vi "TXSIG_Generate(SubVi).vi"(5 "Chip_rate_Threshold":dbl=5.0 format="%#_13g", 7 "ThresHold":dbl=5.0 format="%#_13g", 8 "Version 스위치":bool, 9 "Rc":dbl=5500.0 format="%#_13g", 10 "길이":i32=256, 11 "이름 또는 상대 경로":string) -> (1 "TXN":dbl[](array[numeric]), 2 "TXP":dbl[](array[numeric]), 4 "TXSIG":waveform(dbl)[](graph))   [LabVIEW 2017]
uses:
  <vilib>/Analysis/NI_AALBase.lvlib
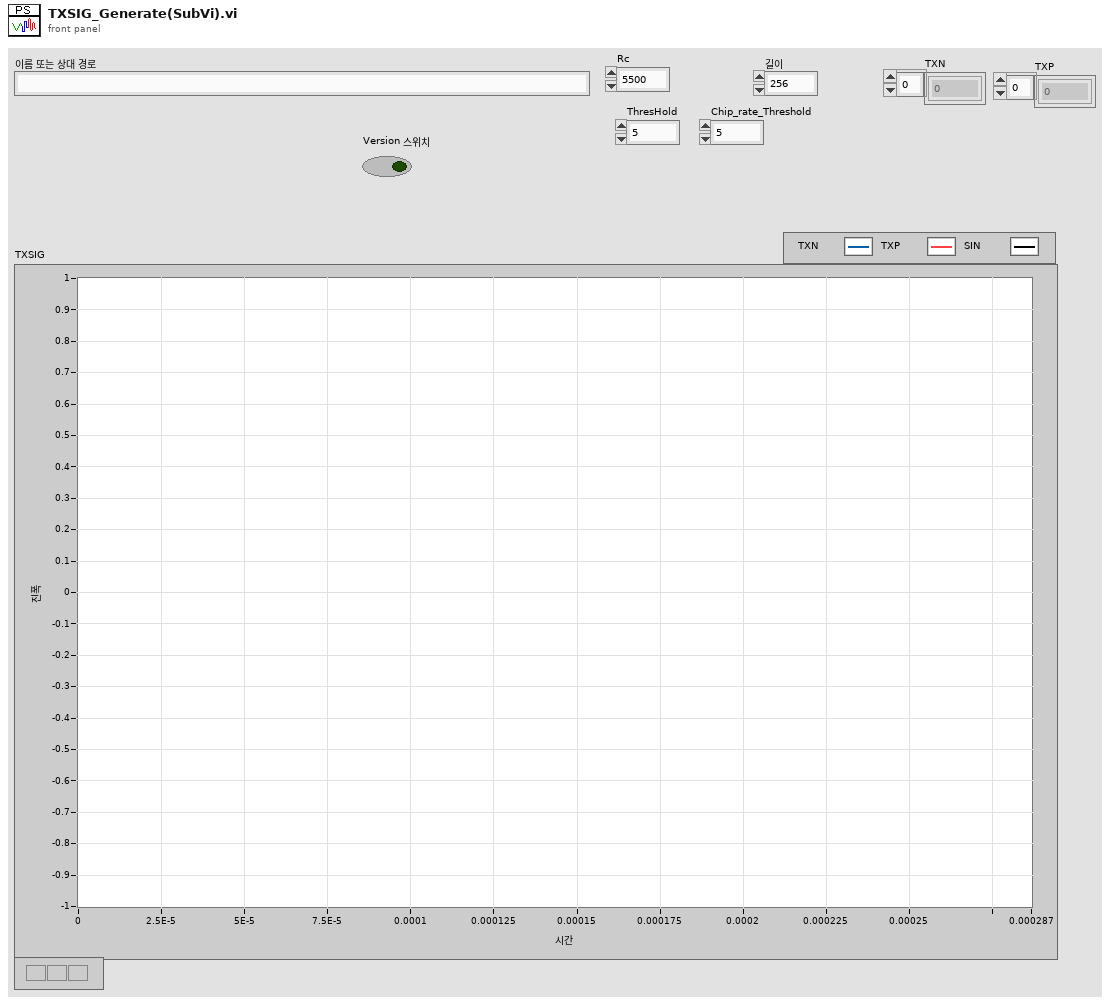
[diagram p1: front panel]
types:
  T1 = enum16{"open", "open or create", "create or replace", "create", "open (read-only)"}
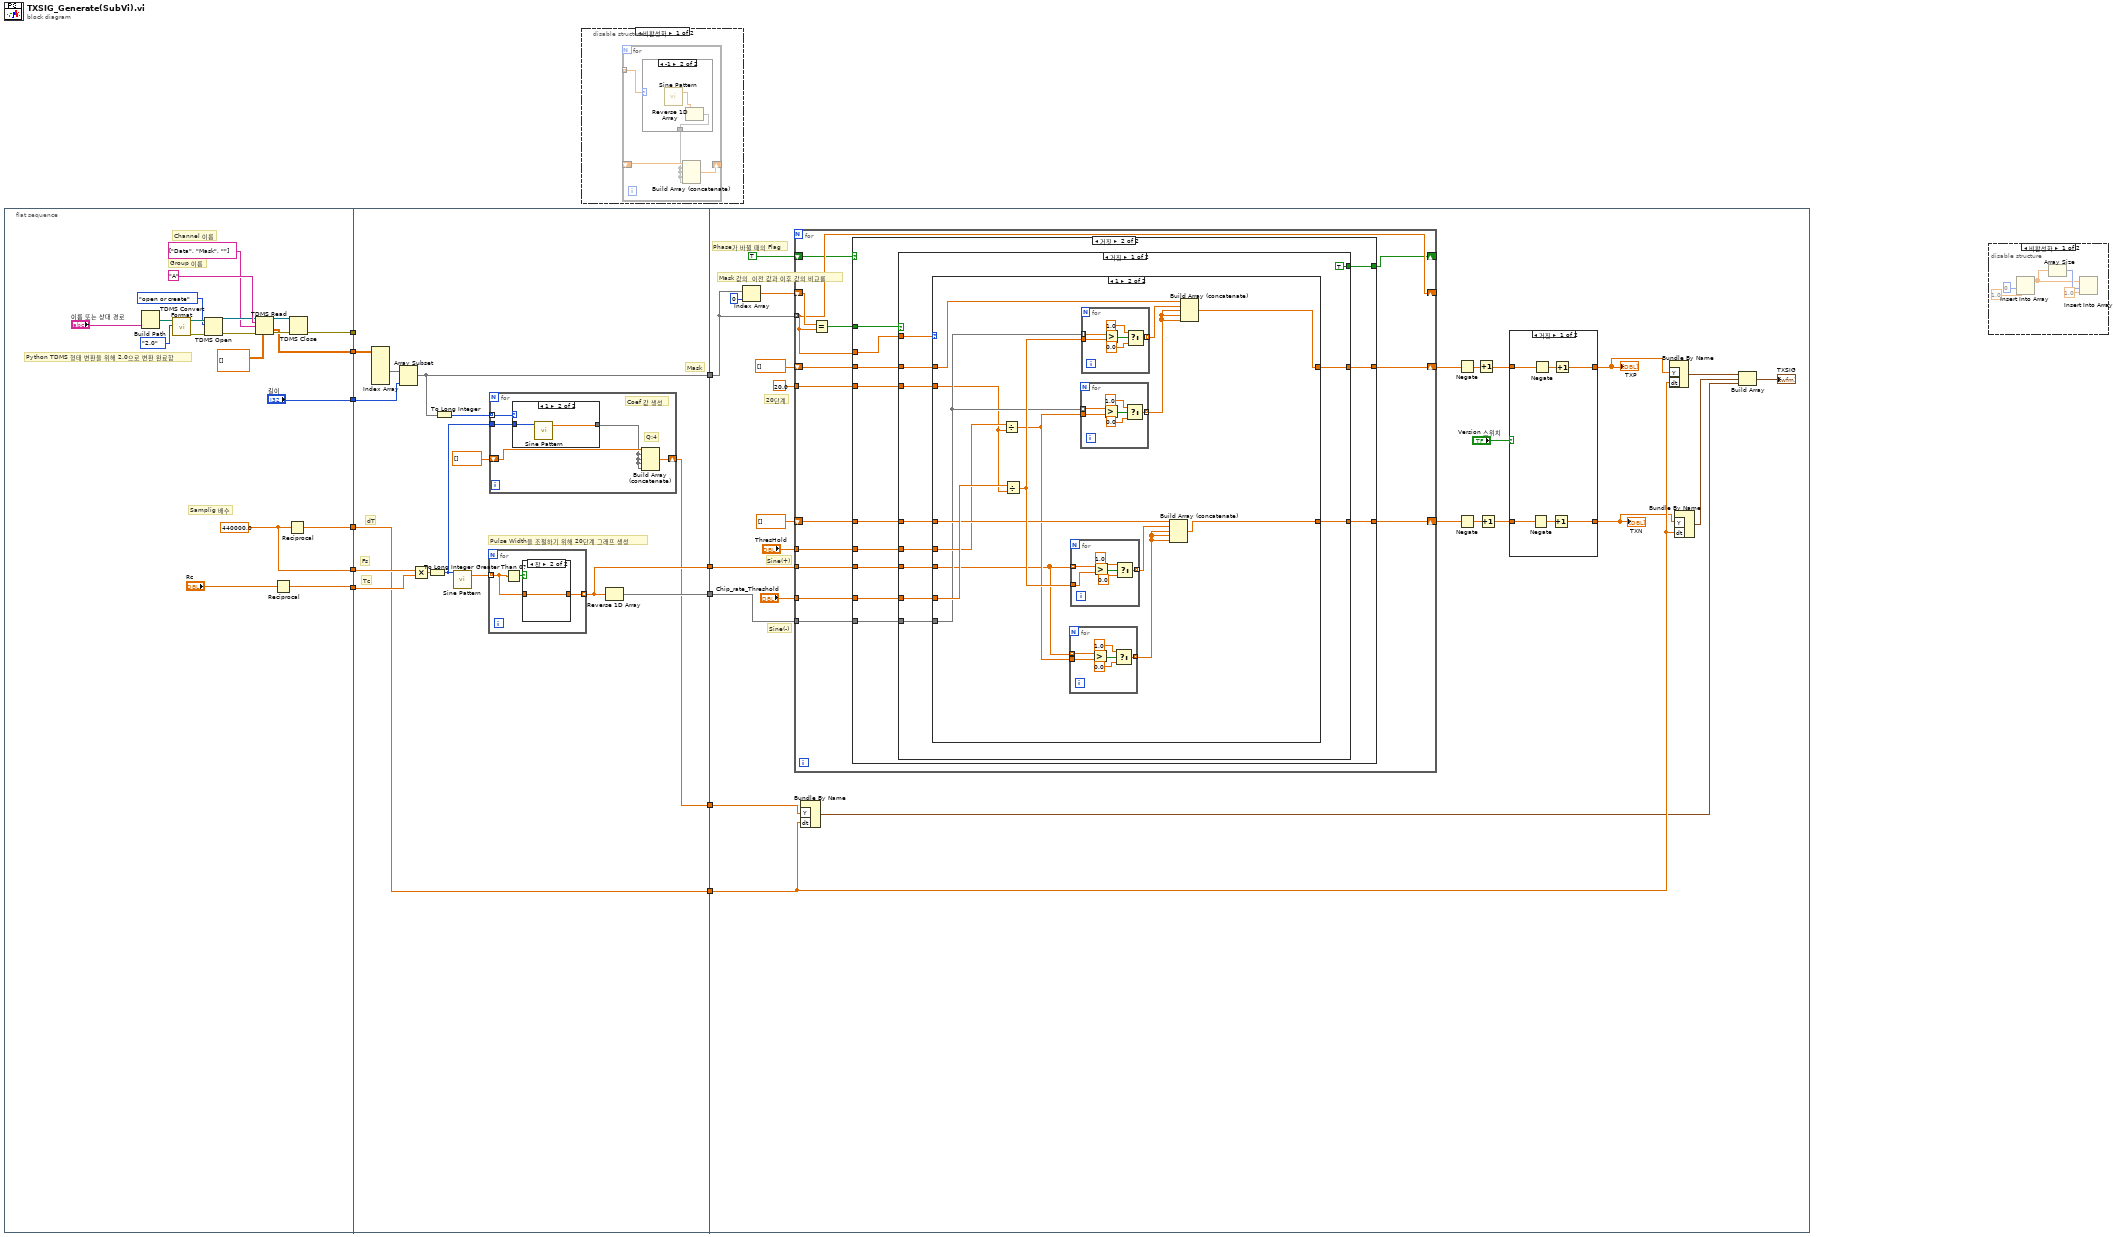
[diagram p0: block diagram]
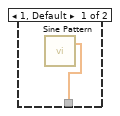
[diagram p2: hidden frame]
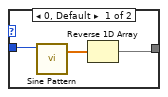
[diagram p5: hidden frame]
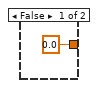
[diagram p6: hidden frame]
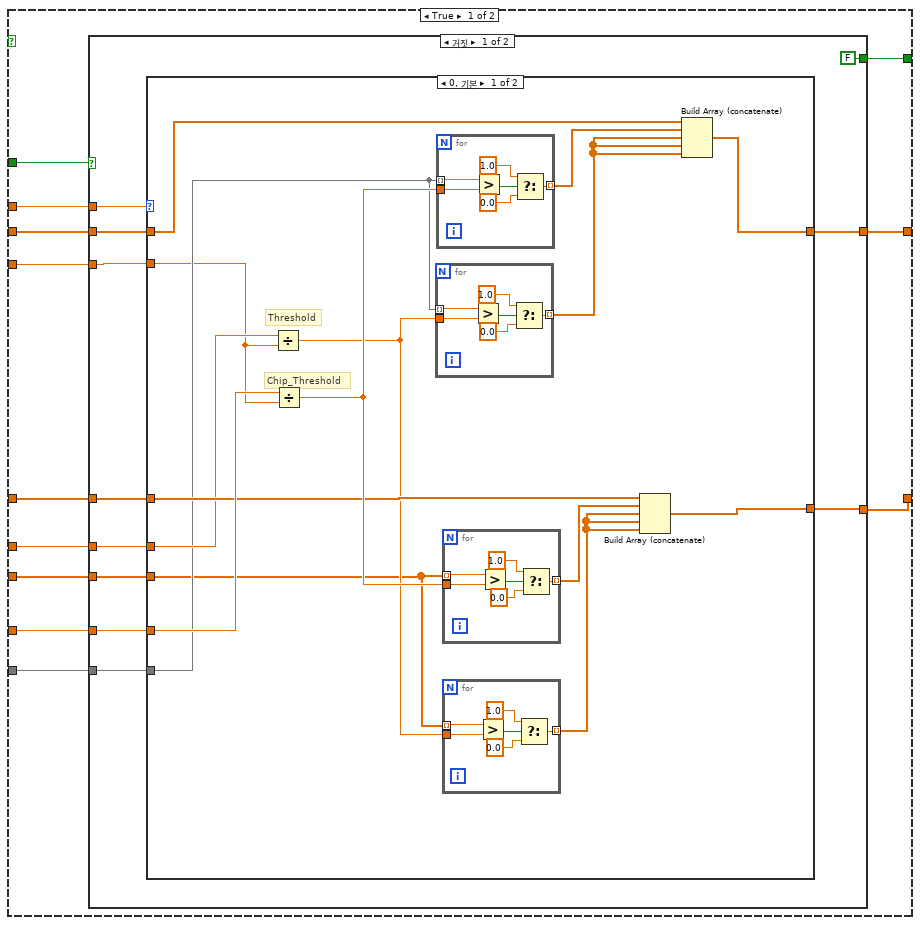
[diagram p8: hidden frame]
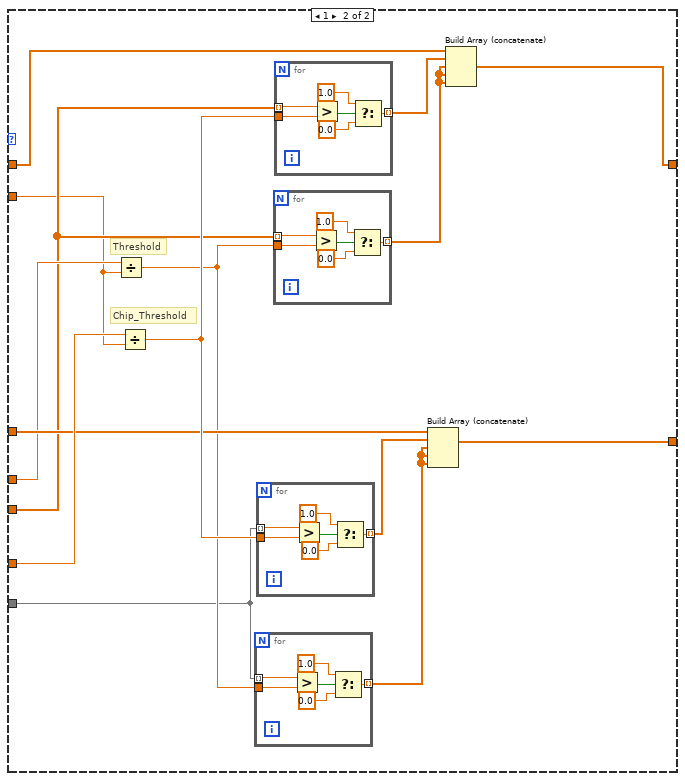
[diagram p9: hidden frame]
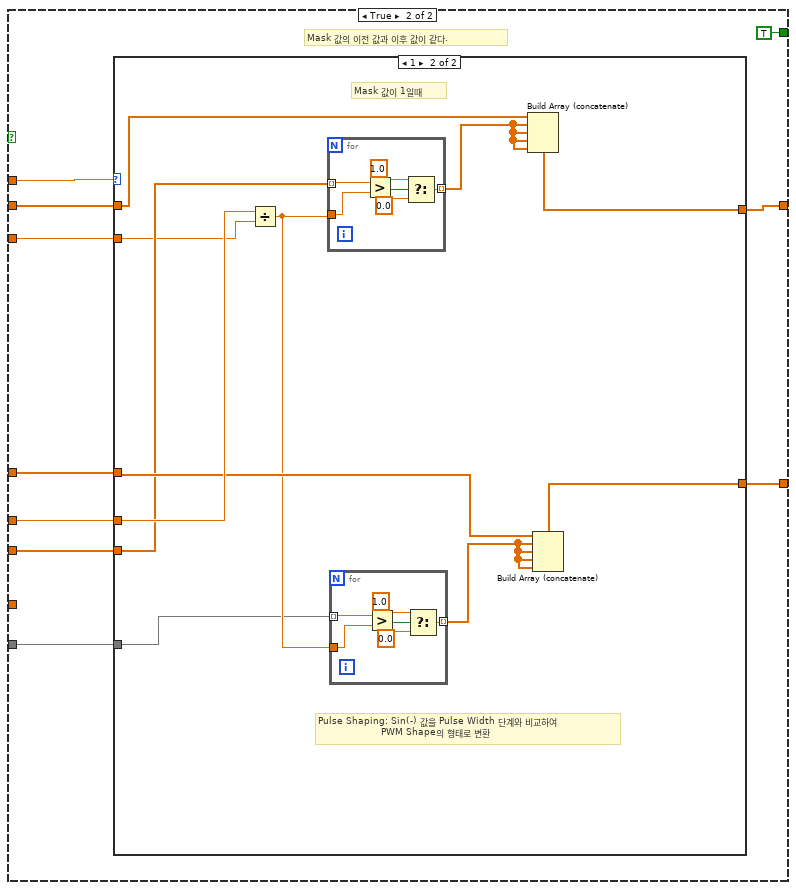
[diagram p10: hidden frame]
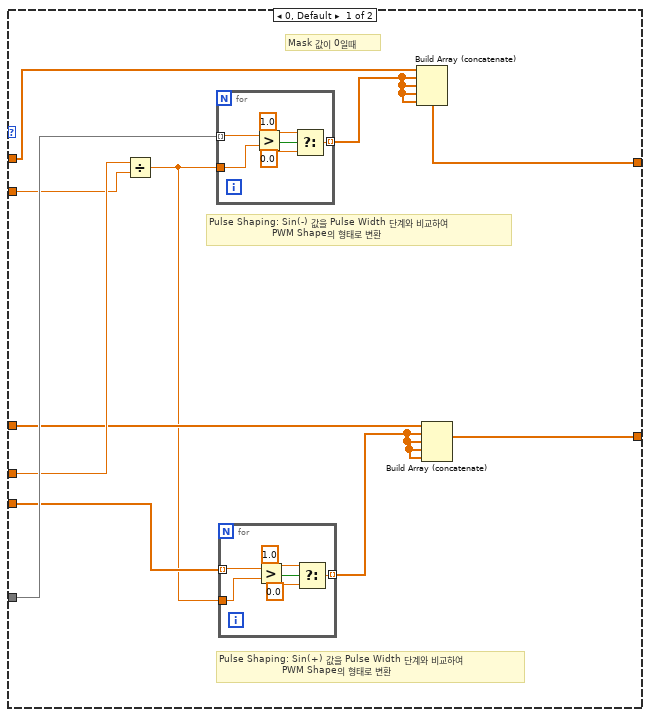
[diagram p11: hidden frame]
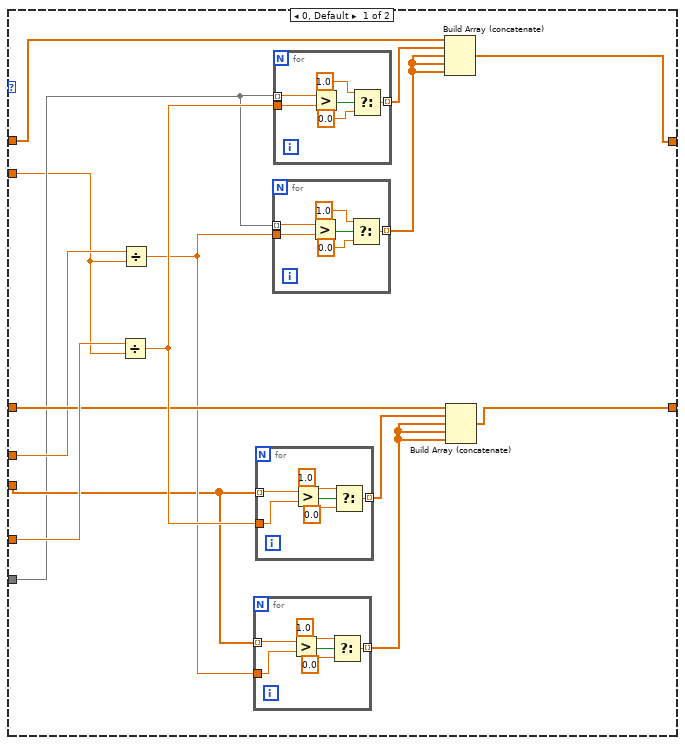
[diagram p12: hidden frame]
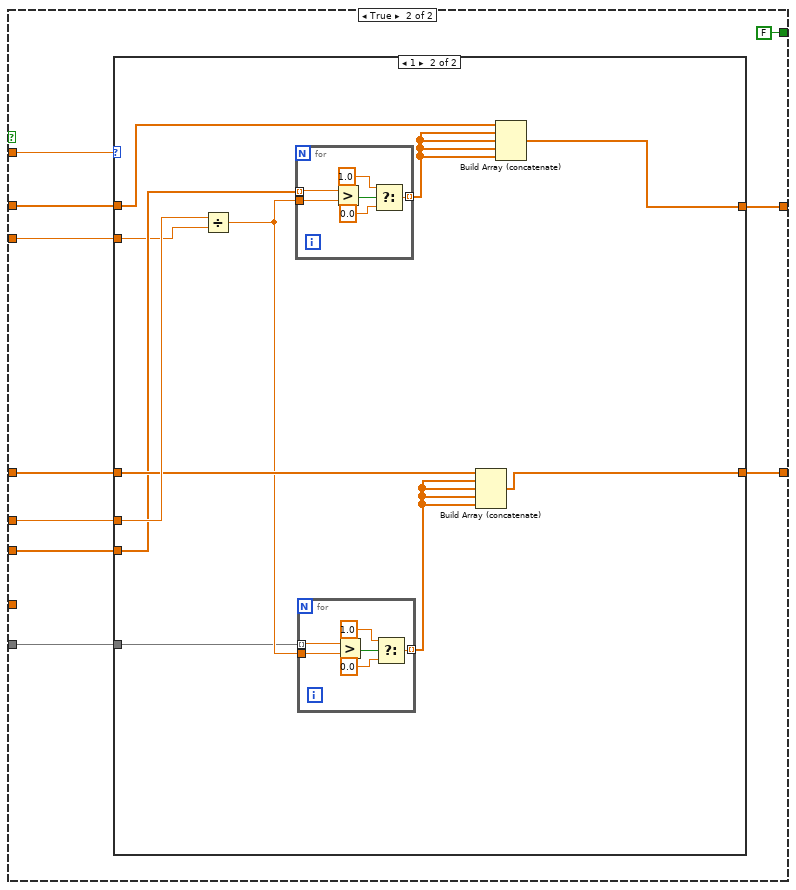
[diagram p13: hidden frame]
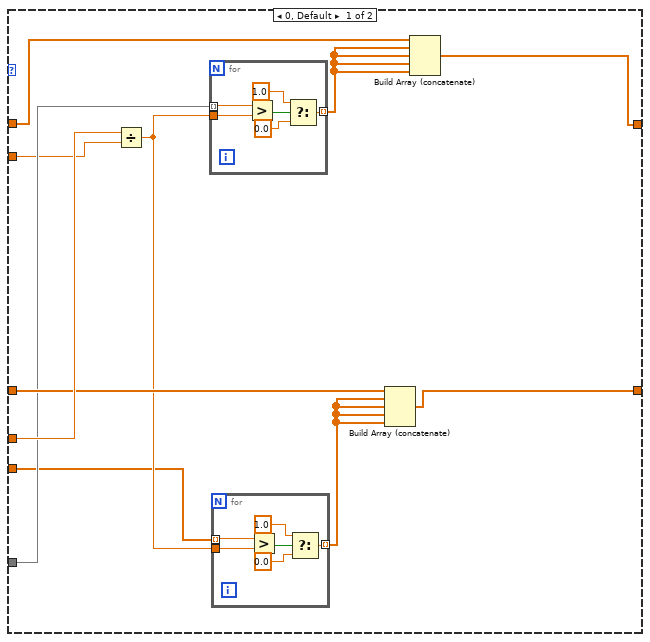
[diagram p14: hidden frame]
diagram:
  n1 = flat-sequence {
    tunnel: [w20] -> w11
    tunnel: [w19] -> w10
    tunnel: ["길이"] -> w6
    tunnel: [w13] -> w5
    tunnel: [w12] -> w4
    tunnel: [w15] -> w3
    tunnel: w10 -> [_]
    tunnel: w11 -> [w43]
    tunnel: [w38] -> w9
    tunnel: [w35] -> w8
    tunnel: [w45] -> w7
    tunnel: w6 -> [w42]
    tunnel: w5 -> [w40]
    tunnel: w4 -> [w39]
    tunnel: w3 -> [w32]
    tunnel: [w34] -> w2
    tunnel: [w32] -> w1
    tunnel: w9 -> [w86]
    tunnel: w8 -> [w83]
    tunnel: w7 -> [w80]
    tunnel: w2 -> [w67]
    tunnel: w1 -> [w72]
    frame #0 {
      w12 = 440000.0
      # "Samplig 배수"
      # "Python TDMS 형태 변환을 위해 2.0으로 변환 완료함"
      # "Group 이름"
      # "Channel 이름"
      n2 = Build Path(name or relative path="이름 또는 상대 경로") -> (appended path=w30:path)  [unwired: 1 in]
      n3 = call <vilib>:"TDMS Convert Format.vi"("target version"=enum16{"1.0", "2.0"}."2.0", "file path"=w30) -> ("error out"=w25:errorcluster, "file path out"=w24:path)  [unwired: 4 in]
      n4 = TDMS Open(8:w25, 10:T1."open or create" ("operation (0:open)"), 11:w24) -> (0:w21:errorcluster, 3:w22:refnum<k34>)  [unwired: 4 in]
      n5 = TDMS Read(0:w22, 5:"A" ("그룹 이름 입력"), 7:string[] ["Data", "Mask", ""] ("채널 이름 입력"), 11:w21, 12:dbl[][] []) -> (4:w27:refnum<k34>, 10:w20:dbl[][], 15:w26:errorcluster)  [unwired: 3 in, 3 out]
      n6 = Reciprocal(x="Rc") -> (1/x=w13:dbl)
      n7 = Reciprocal(x=w12) -> (1/x=w15:dbl)
      n8 = TDMS Close(8:w26, 11:w27) -> (0:w19:errorcluster)  [unwired: 1 out]
    }
    frame #1 {
      # "dT"
      # "Mask"
      # "Pulse Width을 조절하기 위해 20단계 그래프 생성"
      # "Tc"
      # "Fs"
      n9 = Index Array(array=w43) -> (element #2=w44:dbl[])  [unwired: 6 in, 2 out]
      n10 = Array Subset(array=w44, length=w42) -> (w38:dbl[])  [unwired: 1 in]
      n11 = Multiply(x=w39, y=w40) -> (x*y=w41:dbl)
      n12 = To Long Integer(number=w41) -> (32bit integer=w33:i32)
      n13 = To Long Integer(number=w38) -> (32bit integer=w37:i32[])
      n14 = call <vilib>:"Sine Pattern.vi"("samples"=w33) -> ("Sinusoidal Pattern"=w46:dbl[])  [unwired: 3 in, 1 out]
      n15 = for {
        tunnel: w46 -> [w58] mode=indexing
        tunnel: [w57] -> w35 mode=indexing
        n16 = Greater Than 0?(x=w58) -> (x > 0?=w59:bool)
        n17 = case shown="참" w59 {
          tunnel: w58 -> [_ w61]
          tunnel: [0.0 w61] -> w57
          frame False {
          }
          frame True {
          }
        }
      }
      n18 = for {
        tunnel: w33 -> [w51]
        tunnel: w37 -> [w50] mode=indexing
        shift-right: [w47] -> w34
        shift-left: dbl[] [] -> [w49]
        # "Coef 값 생성"
        # "Q:4"
        n19 = case shown="1" w50 {
          tunnel: [w52 w55] -> w48
          tunnel: w51 -> [w54 w56]
          frame 0, Default {
            n20 = call <vilib>:"Sine Pattern.vi"("samples"=w54) -> ("Sinusoidal Pattern"=w53:dbl[])  [unwired: 3 in, 1 out]
            n21 = Reverse 1D Array(array=w53) -> (reversed array=w52:dbl[])
          }
          frame 1 {
            n22 = call <vilib>:"Sine Pattern.vi"("samples"=w56) -> ("Sinusoidal Pattern"=w55:dbl[])  [unwired: 3 in, 1 out]
          }
        }
        n23 = Build Array (concatenate)(w49, w48, w48, w48, w48) -> (w47:dbl[])
      }
      n24 = Reverse 1D Array(array=w35) -> (reversed array=w45:dbl[])
    }
    frame #2 {
      # "20단계"
      # "Mask 값의  이전 값과 이후 값의 비교를"
      # "Phase가 바뀔 때의 Flag"
      # "Sine(-)"
      # "Sine(+)"
      n25 = Index Array(array=w86, index=0 ("인덱스")) -> (element=w84:dbl)
      n26 = for {
        shift-right: [w97] -> _
        shift-left: TRUE -> [w98]
        tunnel: w86 -> [w107] mode=indexing
        shift-right: [w107] -> _
        shift-left: w84 -> [w109]
        tunnel: w83 -> [w106]
        shift-right: [w102] -> w77
        shift-left: dbl[] [] -> [w104]
        shift-right: [w101] -> w76
        shift-left: dbl[] [] -> [w105]
        tunnel: w80 -> [w103]
        tunnel: "ThresHold" -> [w100]
        tunnel: "Chip_rate_Threshold" -> [w99]
        tunnel: 20.0 ("y") -> [w96]
        n27 = Equal?(x=w109, y=w107) -> (x = y?=w108:bool)
        n28 = case shown="거짓" w98 {
          tunnel: w108 -> [w121 w278]
          tunnel: w107 -> [w120 w277]
          tunnel: w106 -> [w119 w276]
          tunnel: w105 -> [w118 w275]
          tunnel: w104 -> [w117 w274]
          tunnel: w103 -> [w116 w273]
          tunnel: [w115 w272] -> w102
          tunnel: [w114 w271] -> w101
          tunnel: w100 -> [w113 w270]
          tunnel: w99 -> [w112 w269]
          tunnel: [w111 w268] -> w97
          tunnel: w96 -> [w110 w267]
          frame True {
            n29 = case shown="거짓" w121 {
              tunnel: w120 -> [w132 w220]
              tunnel: w119 -> [w128 w216]
              tunnel: w118 -> [w130 w219]
              tunnel: w117 -> [w131 w218]
              tunnel: w116 -> [w127 w217]
              tunnel: [w125 w215] -> w115
              tunnel: [w124 w214] -> w114
              tunnel: w113 -> [w129 w213]
              tunnel: w112 -> [w126 _]
              tunnel: [FALSE TRUE] -> w111
              tunnel: w110 -> [w122 w211]
              frame False {
                n30 = case shown="0, 기본" w132 {
                  tunnel: w131 -> [w147 w186]
                  tunnel: w130 -> [w143 w182]
                  tunnel: w129 -> [w139 w178]
                  tunnel: w128 -> [w135 w174]
                  tunnel: w127 -> [w138 w173]
                  tunnel: w126 -> [w146 w185]
                  tunnel: [w145 w184] -> w125
                  tunnel: [w142 w181] -> w124
                  tunnel: w122 -> [w133 w172]
                  frame 0, Default {
                    # "Threshold"
                    # "Chip_Threshold"
                    n31 = Divide(x=w139, y=w133) -> (x/y=w136:dbl)
                    n32 = Divide(x=w146, y=w133) -> (x/y=w144:dbl)
                    n33 = for {
                      tunnel: w138 -> [w159] mode=indexing
                      tunnel: w136 -> [w158]
                      tunnel: [w154] -> w137 mode=indexing
                      n34 = Greater?(x=w159, y=w158) -> (0:w157:bool)
                      n35 = Select(t=1.0, s=w157, f=0.0) -> (s? t:f=w154:dbl)
                    }
                    n36 = for {
                      tunnel: w138 -> [w171] mode=indexing
                      tunnel: w144 -> [w170]
                      tunnel: [w166] -> w141 mode=indexing
                      n37 = Greater?(x=w171, y=w170) -> (0:w169:bool)
                      n38 = Select(t=1.0, s=w169, f=0.0) -> (s? t:f=w166:dbl)
                    }
                    n39 = for {
                      tunnel: w135 -> [w165] mode=indexing
                      tunnel: w144 -> [w164]
                      tunnel: [w160] -> w140 mode=indexing
                      n40 = Greater?(x=w165, y=w164) -> (0:w163:bool)
                      n41 = Select(t=1.0, s=w163, f=0.0) -> (s? t:f=w160:dbl)
                    }
                    n42 = for {
                      tunnel: w135 -> [w153] mode=indexing
                      tunnel: w136 -> [w152]
                      tunnel: [w148] -> w134 mode=indexing
                      n43 = Greater?(x=w153, y=w152) -> (0:w151:bool)
                      n44 = Select(t=1.0, s=w151, f=0.0) -> (s? t:f=w148:dbl)
                    }
                    n45 = Build Array (concatenate)(w143, w140, w134, w134, w134) -> (w142:dbl[])
                    n46 = Build Array (concatenate)(w147, w141, w137, w137, w137) -> (w145:dbl[])
                  }
                  frame 1 {
                    # "Chip_Threshold"
                    # "Threshold"
                    n47 = Divide(x=w178, y=w172) -> (x/y=w176:dbl)
                    n48 = Divide(x=w185, y=w172) -> (x/y=w183:dbl)
                    n49 = for {
                      tunnel: w173 -> [w192] mode=indexing
                      tunnel: w176 -> [w191]
                      tunnel: [w187] -> w175 mode=indexing
                      n50 = Greater?(x=w192, y=w191) -> (0:w190:bool)
                      n51 = Select(t=1.0, s=w190, f=0.0) -> (s? t:f=w187:dbl)
                    }
                    n52 = for {
                      tunnel: w173 -> [w204] mode=indexing
                      tunnel: w183 -> [w203]
                      tunnel: [w199] -> w179 mode=indexing
                      n53 = Greater?(x=w204, y=w203) -> (0:w202:bool)
                      n54 = Select(t=1.0, s=w202, f=0.0) -> (s? t:f=w199:dbl)
                    }
                    n55 = for {
                      tunnel: w174 -> [w198] mode=indexing
                      tunnel: w176 -> [w197]
                      tunnel: [w193] -> w177 mode=indexing
                      n56 = Greater?(x=w198, y=w197) -> (0:w196:bool)
                      n57 = Select(t=1.0, s=w196, f=0.0) -> (s? t:f=w193:dbl)
                    }
                    n58 = for {
                      tunnel: w174 -> [w210] mode=indexing
                      tunnel: w183 -> [w209]
                      tunnel: [w205] -> w180 mode=indexing
                      n59 = Greater?(x=w210, y=w209) -> (0:w208:bool)
                      n60 = Select(t=1.0, s=w208, f=0.0) -> (s? t:f=w205:dbl)
                    }
                    n61 = Build Array (concatenate)(w182, w179, w175, w175, w175) -> (w181:dbl[])
                    n62 = Build Array (concatenate)(w186, w180, w177, w177, w177) -> (w184:dbl[])
                  }
                }
              }
              frame True {
                # "Mask 값의 이전 값과 이후 값이 같다."
                n63 = case shown="1" w220 {
                  tunnel: w219 -> [w227 w251]
                  tunnel: w218 -> [w231 w254]
                  tunnel: w217 -> [w229 w246]
                  tunnel: w216 -> [w226 w245]
                  tunnel: [w230 w253] -> w215
                  tunnel: [w224 w249] -> w214
                  tunnel: w213 -> [w228 w252]
                  tunnel: w211 -> [w221 w244]
                  frame 0, Default {
                    # "Pulse Shaping: Sin(+) 값을 Pulse Width 단계와 비교하여\n                     PWM Shape의 형태로 변환"
                    # "Pulse Shaping: Sin(-) 값을 Pulse Width 단계와 비교하여\n                     PWM Shape의 형태로 변환"
                    # "Mask 값이 0일때"
                    n64 = Divide(x=w228, y=w221) -> (x/y=w225:dbl)
                    n65 = for {
                      tunnel: w229 -> [w243] mode=indexing
                      tunnel: w225 -> [w242]
                      tunnel: [w238] -> w223 mode=indexing
                      n66 = Greater?(x=w243, y=w242) -> (0:w241:bool)
                      n67 = Select(t=1.0, s=w241, f=0.0) -> (s? t:f=w238:dbl)
                    }
                    n68 = for {
                      tunnel: w226 -> [w237] mode=indexing
                      tunnel: w225 -> [w236]
                      tunnel: [w232] -> w222 mode=indexing
                      n69 = Greater?(x=w237, y=w236) -> (0:w235:bool)
                      n70 = Select(t=1.0, s=w235, f=0.0) -> (s? t:f=w232:dbl)
                    }
                    n71 = Build Array (concatenate)(w231, w223, w223, w223, w223) -> (w230:dbl[])
                    n72 = Build Array (concatenate)(w227, w222, w222, w222, w222) -> (w224:dbl[])
                  }
                  frame 1 {
                    # "Pulse Shaping: Sin(-) 값을 Pulse Width 단계와 비교하여\n                     PWM Shape의 형태로 변환"
                    # "Mask 값이 1일때"
                    n73 = Divide(x=w252, y=w244) -> (x/y=w250:dbl)
                    n74 = for {
                      tunnel: w245 -> [w266] mode=indexing
                      tunnel: w250 -> [w265]
                      tunnel: [w261] -> w248 mode=indexing
                      n75 = Greater?(x=w266, y=w265) -> (0:w264:bool)
                      n76 = Select(t=1.0, s=w264, f=0.0) -> (s? t:f=w261:dbl)
                    }
                    n77 = for {
                      tunnel: w246 -> [w260] mode=indexing
                      tunnel: w250 -> [w259]
                      tunnel: [w255] -> w247 mode=indexing
                      n78 = Greater?(x=w260, y=w259) -> (0:w258:bool)
                      n79 = Select(t=1.0, s=w258, f=0.0) -> (s? t:f=w255:dbl)
                    }
                    n80 = Build Array (concatenate)(w254, w248, w248, w248, w248) -> (w253:dbl[])
                    n81 = Build Array (concatenate)(w251, w247, w247, w247, w247) -> (w249:dbl[])
                  }
                }
              }
            }
          }
          frame False {
            n82 = case shown="거짓" w278 {
              tunnel: w277 -> [w289 w377]
              tunnel: w276 -> [w285 w373]
              tunnel: w275 -> [w287 w376]
              tunnel: w274 -> [w288 w375]
              tunnel: w273 -> [w284 w374]
              tunnel: [w282 w372] -> w272
              tunnel: [w281 w371] -> w271
              tunnel: w270 -> [w286 w370]
              tunnel: w269 -> [w283 _]
              tunnel: [TRUE FALSE] -> w268
              tunnel: w267 -> [w279 w368]
              frame False {
                n83 = case shown="1" w289 {
                  tunnel: w288 -> [w304 w343]
                  tunnel: w287 -> [w300 w339]
                  tunnel: w286 -> [w296 w335]
                  tunnel: w285 -> [w293 w330]
                  tunnel: w284 -> [w292 w331]
                  tunnel: w283 -> [w303 w342]
                  tunnel: [w302 w341] -> w282
                  tunnel: [w299 w338] -> w281
                  tunnel: w279 -> [w291 w329]
                  frame 0, Default {
                    n84 = Divide(x=w303, y=w291) -> (x/y=w301:dbl)
                    n85 = Divide(x=w296, y=w291) -> (x/y=w294:dbl)
                    n86 = for {
                      tunnel: w293 -> [w310] mode=indexing
                      tunnel: w294 -> [w309]
                      tunnel: [w305] -> w290 mode=indexing
                      n87 = Greater?(x=w310, y=w309) -> (0:w308:bool)
                      n88 = Select(t=1.0, s=w308, f=0.0) -> (s? t:f=w305:dbl)
                    }
                    n89 = for {
                      tunnel: w293 -> [w322] mode=indexing
                      tunnel: w301 -> [w321]
                      tunnel: [w317] -> w297 mode=indexing
                      n90 = Greater?(x=w322, y=w321) -> (0:w320:bool)
                      n91 = Select(t=1.0, s=w320, f=0.0) -> (s? t:f=w317:dbl)
                    }
                    n92 = for {
                      tunnel: w292 -> [w316] mode=indexing
                      tunnel: w294 -> [w315]
                      tunnel: [w311] -> w295 mode=indexing
                      n93 = Greater?(x=w316, y=w315) -> (0:w314:bool)
                      n94 = Select(t=1.0, s=w314, f=0.0) -> (s? t:f=w311:dbl)
                    }
                    n95 = for {
                      tunnel: w292 -> [w328] mode=indexing
                      tunnel: w301 -> [w327]
                      tunnel: [w323] -> w298 mode=indexing
                      n96 = Greater?(x=w328, y=w327) -> (0:w326:bool)
                      n97 = Select(t=1.0, s=w326, f=0.0) -> (s? t:f=w323:dbl)
                    }
                    n98 = Build Array (concatenate)(w304, w298, w295, w295, w295) -> (w302:dbl[])
                    n99 = Build Array (concatenate)(w300, w297, w290, w290, w290) -> (w299:dbl[])
                  }
                  frame 1 {
                    n100 = Divide(x=w335, y=w329) -> (x/y=w333:dbl)
                    n101 = Divide(x=w342, y=w329) -> (x/y=w340:dbl)
                    n102 = for {
                      tunnel: w330 -> [w349] mode=indexing
                      tunnel: w333 -> [w348]
                      tunnel: [w344] -> w332 mode=indexing
                      n103 = Greater?(x=w349, y=w348) -> (0:w347:bool)
                      n104 = Select(t=1.0, s=w347, f=0.0) -> (s? t:f=w344:dbl)
                    }
                    n105 = for {
                      tunnel: w330 -> [w361] mode=indexing
                      tunnel: w340 -> [w360]
                      tunnel: [w356] -> w336 mode=indexing
                      n106 = Greater?(x=w361, y=w360) -> (0:w359:bool)
                      n107 = Select(t=1.0, s=w359, f=0.0) -> (s? t:f=w356:dbl)
                    }
                    n108 = for {
                      tunnel: w331 -> [w355] mode=indexing
                      tunnel: w333 -> [w354]
                      tunnel: [w350] -> w334 mode=indexing
                      n109 = Greater?(x=w355, y=w354) -> (0:w353:bool)
                      n110 = Select(t=1.0, s=w353, f=0.0) -> (s? t:f=w350:dbl)
                    }
                    n111 = for {
                      tunnel: w331 -> [w367] mode=indexing
                      tunnel: w340 -> [w366]
                      tunnel: [w362] -> w337 mode=indexing
                      n112 = Greater?(x=w367, y=w366) -> (0:w365:bool)
                      n113 = Select(t=1.0, s=w365, f=0.0) -> (s? t:f=w362:dbl)
                    }
                    n114 = Build Array (concatenate)(w339, w336, w332, w332, w332) -> (w338:dbl[])
                    n115 = Build Array (concatenate)(w343, w337, w334, w334, w334) -> (w341:dbl[])
                  }
                }
              }
              frame True {
                n116 = case shown="1" w377 {
                  tunnel: w376 -> [w385 w408]
                  tunnel: w375 -> [w388 w411]
                  tunnel: w374 -> [w380 w403]
                  tunnel: w373 -> [w379 w402]
                  tunnel: [w387 w410] -> w372
                  tunnel: [w383 w406] -> w371
                  tunnel: w370 -> [w386 w409]
                  tunnel: w368 -> [w378 w401]
                  frame 0, Default {
                    n117 = Divide(x=w386, y=w378) -> (x/y=w384:dbl)
                    n118 = for {
                      tunnel: w380 -> [w400] mode=indexing
                      tunnel: w384 -> [w399]
                      tunnel: [w395] -> w382 mode=indexing
                      n119 = Greater?(x=w400, y=w399) -> (0:w398:bool)
                      n120 = Select(t=1.0, s=w398, f=0.0) -> (s? t:f=w395:dbl)
                    }
                    n121 = for {
                      tunnel: w379 -> [w394] mode=indexing
                      tunnel: w384 -> [w393]
                      tunnel: [w389] -> w381 mode=indexing
                      n122 = Greater?(x=w394, y=w393) -> (0:w392:bool)
                      n123 = Select(t=1.0, s=w392, f=0.0) -> (s? t:f=w389:dbl)
                    }
                    n124 = Build Array (concatenate)(w385, w381, w381, w381, w381) -> (w383:dbl[])
                    n125 = Build Array (concatenate)(w388, w382, w382, w382, w382) -> (w387:dbl[])
                  }
                  frame 1 {
                    n126 = Divide(x=w409, y=w401) -> (x/y=w407:dbl)
                    n127 = for {
                      tunnel: w402 -> [w423] mode=indexing
                      tunnel: w407 -> [w422]
                      tunnel: [w418] -> w405 mode=indexing
                      n128 = Greater?(x=w423, y=w422) -> (0:w421:bool)
                      n129 = Select(t=1.0, s=w421, f=0.0) -> (s? t:f=w418:dbl)
                    }
                    n130 = for {
                      tunnel: w403 -> [w417] mode=indexing
                      tunnel: w407 -> [w416]
                      tunnel: [w412] -> w404 mode=indexing
                      n131 = Greater?(x=w417, y=w416) -> (0:w415:bool)
                      n132 = Select(t=1.0, s=w415, f=0.0) -> (s? t:f=w412:dbl)
                    }
                    n133 = Build Array (concatenate)(w408, w404, w404, w404, w404) -> (w406:dbl[])
                    n134 = Build Array (concatenate)(w411, w405, w405, w405, w405) -> (w410:dbl[])
                  }
                }
              }
            }
          }
        }
      }
      n135 = Bundle By Name("Y"=w67, "dt"=w72) -> (w69:waveform(dbl))  [unwired: 1 in]
      n136 = Negate(x=w77) -> (-x=w75:dbl[])
      n137 = Negate(x=w76) -> (-x=w74:dbl[])
      n138 = Increment(x=w75) -> (x+1=w65:dbl[])
      n139 = Increment(x=w74) -> (x+1=w63:dbl[])
      n140 = case shown="거짓" "Version 스위치" {
        tunnel: [w90 w95] -> w64
        tunnel: w65 -> [w93 w95]
        tunnel: [w88 w94] -> w62
        tunnel: w63 -> [w92 w94]
        frame False {
          n141 = Negate(x=w92) -> (-x=w89:dbl[])
          n142 = Negate(x=w93) -> (-x=w91:dbl[])
          n143 = Increment(x=w89) -> (x+1=w88:dbl[])
          n144 = Increment(x=w91) -> (x+1=w90:dbl[])
        }
        frame True {
        }
      }
      "TXP" <- w64
      "TXN" <- w62
      n145 = Bundle By Name("Y"=w64, "dt"=w72) -> (w71:waveform(dbl))  [unwired: 1 in]
      n146 = Bundle By Name("Y"=w62, "dt"=w72) -> (w70:waveform(dbl))  [unwired: 1 in]
      n147 = Build Array(w71, w70, w69) -> (→"TXSIG":waveform(dbl)[])
    }
  }
  n148 = disable-structure shown="비활성화" {
    frame Disabled {
      n149 = for {
        tunnel: _ -> [w427] mode=indexing
        shift-right: [w425] -> _
        shift-left: _ -> [w426]
        n150 = case shown="-1" w427 {
          tunnel: [w428 w429] -> w424
          frame 1, Default {
            n151 = call <vilib>:"Sine Pattern.vi"() -> ("Sinusoidal Pattern"=w428:dbl[])  [unwired: 4 in, 1 out]
          }
          frame -1 {
            n152 = call <vilib>:"Sine Pattern.vi"() -> ("Sinusoidal Pattern"=w430:dbl[])  [unwired: 4 in, 1 out]
            n153 = Reverse 1D Array(array=w430) -> (reversed array=w429:dbl[])
          }
        }
        n154 = Build Array (concatenate)(w426, w424, w424, w424, w424) -> (w425:dbl[])
      }
    }
    frame Enabled {
    }
  }
  n155 = disable-structure shown="비활성화" {
    frame Disabled {
      n156 = Insert Into Array(index=0 ("인덱스"), new element=1.0 ("새 원소/부분배열")) -> (w433:dbl[])  [unwired: 1 in]
      n157 = Array Size(array=w433) -> (size(s)=w434:i32)
      n158 = Insert Into Array(array=w433, index=w434, new element=1.0 ("새 원소/부분배열")) -> ()  [unwired: 1 out]
    }
    frame Enabled {
    }
  }
